vi "Tester.vi"() -> ()   [LabVIEW 2015]
uses:
  <resource>/Framework/Providers/lveio/public/EIOExtName.ctl
  <resource>/Framework/Providers/lveio/private/EIOResName.ctl
  <resource>/Framework/Providers/lveio/public/EIOResourceTree_TargetItem_GetProperty.vi
  <resource>/Framework/Providers/lveio/private/EIOResourceTree_TargetItem_GetResources.vi
  <resource>/Framework/Providers/lveio/public/EIOResourceTree_ProjectItem_GetDescendantNames.vi
panel:
  out "resources":T1[](array[typedef])
  out "value 2":string
  out "Array 3":string[](array[string])
  out "names":T2[](array[typedef])
  out "Tag:Get Names":string[](array[string])
  out "Array 2":string[](array[string])
  out "Array":string[](array[string])
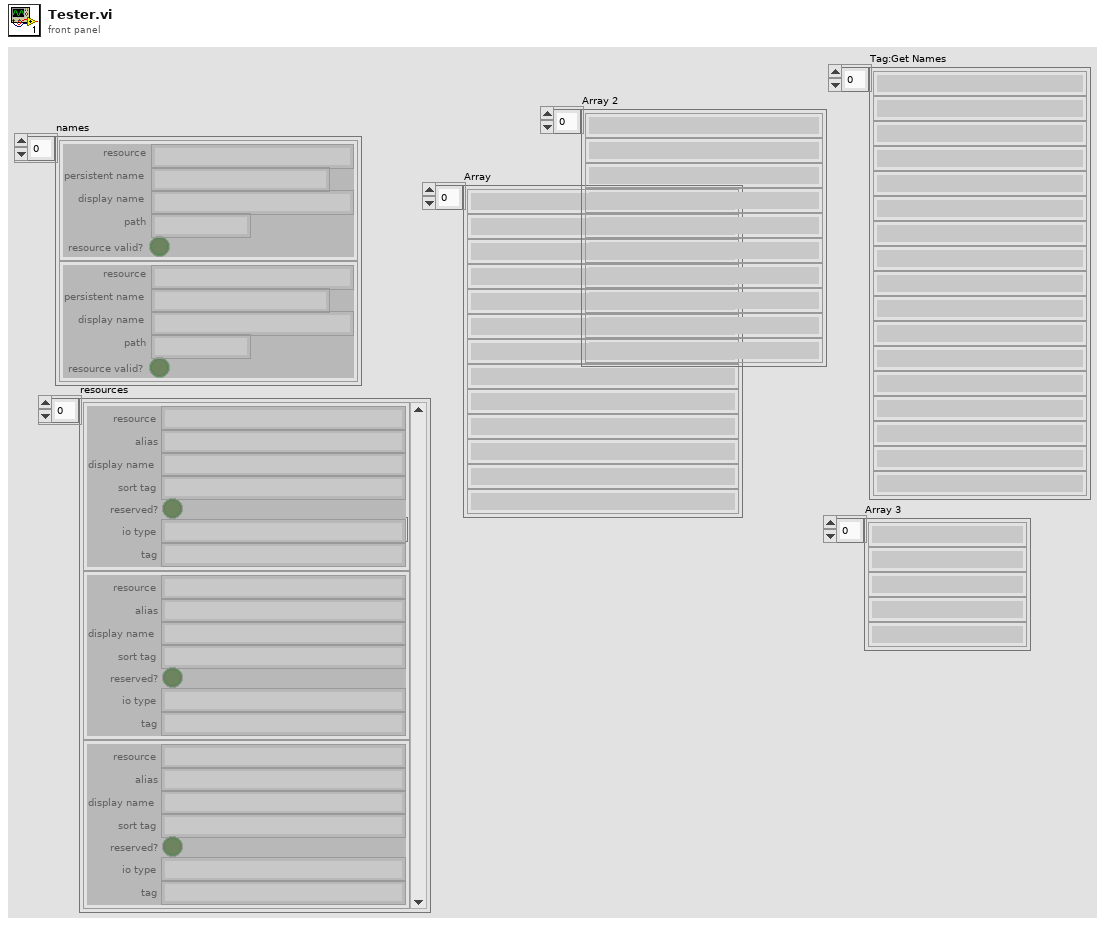
[diagram p1: front panel]
types:
  T1 = typedef "EIOResName.ctl" = cluster{"resource":string, "alias":string, "display name":string, "sort tag":string, "reserved?":bool, "io type":string, "tag":string}
  T2 = typedef "EIOExtName.ctl" = cluster{"resource":string, "persistent name":string, "display name":string, "path":string, "resource valid?":bool}
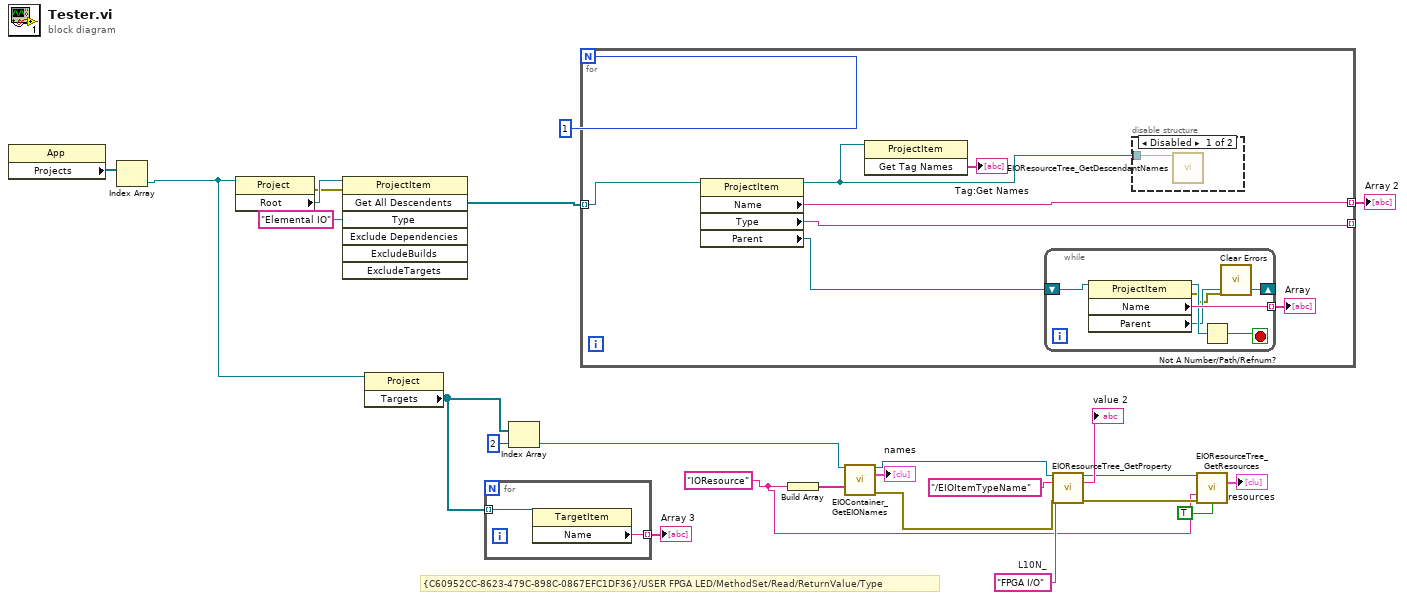
[diagram p0: block diagram]
diagram:
  w9 = "FPGA I/O"  # L10N_
  w3 = "IOResource" ("protocol")
  # "{C60952CC-8623-479C-898C-0867EFC1DF36}/USER FPGA LED/MethodSet/Read/ReturnValue/Type"
  n1 = property class="App"() -> ("Projects"=w24:refnum<vi>[])  [unwired: 2 in, 2 out]
  n2 = Index Array(array=w24) -> (element=w17:refnum<vi>)  [unwired: 1 in]
  n3 = property class="Project"(reference=w17) -> (error out=w22:errorcluster, "Root"=w23:refnum<vi>)  [unwired: 1 in, 1 out]
  n4 = invoke class="ProjectItem" method="Get All Descendents"(reference=w23, error in=w22, "Type"="Elemental IO") -> ("All Descendents"=w20:refnum<vi>[])  [unwired: 4 in, 6 out]
  n5 = property class="Project"(reference=w17) -> ("Targets"=w13:refnum<vi>[])  [unwired: 1 in, 2 out]
  n6 = for {
    tunnel: w13 -> [w26] mode=indexing
    tunnel: [w25] -> w11 mode=indexing
    n7 = property class="TargetItem"(reference=w26) -> ("Name"=w25:string)  [unwired: 1 in, 2 out]
  }
  "Array 3" <- w11
  n8 = Index Array(array=w13, index=2) -> (element=w12:refnum<vi>)
  n9 = for {
    N: 1 -> [_]
    tunnel: w20 -> [w33] mode=indexing
    tunnel: [w32] -> w18 mode=indexing
    tunnel: [w31] -> _ mode=indexing
    n10 = property class="ProjectItem"(reference=w33) -> (reference out=w28:refnum<vi>, "Name"=w32:string, "Type"=w31:string, "Parent"=w30:refnum<vi>)  [unwired: 1 in, 1 out]
    n11 = invoke class="ProjectItem" method="Get Tag Names"(reference=w28) -> ("Get Tag Names"=→"Tag:Get Names":string[])  [unwired: 2 in, 2 out]
    n12 = while {
      tunnel: [w39] -> w29 mode=indexing
      shift-right: [w36] -> _
      shift-left: w30 -> [w40]
      stop <- w37 stop-if-true
      n13 = property class="ProjectItem"(reference=w40) -> (reference out=w38:refnum<vi>, error out=w35:errorcluster, "Name"=w39:string, "Parent"=w36:refnum<vi>)  [unwired: 1 in]
      n14 = Not A Number/Path/Refnum?(number/path/refnum=w38) -> (NaN/Path/Refnum?=w37:bool)
      n15 = call <vilib>:"Clear Errors.vi"("error in (no error)"=w35) -> ()  [unwired: 5 in, 2 out]
    }
    "Array" <- w29
    n16 = disable-structure shown="Disabled" {
      disable-tunnel: w28 -> [w34 _]
      frame Disabled {
        n17 = call-poly <resource>:"EIOResourceTree_GetDescendantNames.vi"("Refnum In"=w34) -> ()  [unwired: 3 in, 12 out]
      }
      frame Enabled {
      }
    }
  }
  "Array 2" <- w18
  n18 = Build Array(w3) -> (w15:string[])
  n19 = call <resource>:"EIOContainer_GetEIONames.vi"("TargetItem Refnum In"=w12, "include protocols"=w15) -> ("TargetItem Refnum Out"=w8:refnum<vi>, "names"=→"names":T2[], "error out"=w7:errorcluster)  [unwired: 2 in, 9 out]
  n20 = call-poly <resource>:"EIOResourceTree_GetProperty.vi"("Refnum In"=w8, "property"="/EIOItemTypeName", "default value"=w9, "error in (no error)"=w7) -> ("Refnum Out"=w5:refnum<vi>, "value"=→"value 2":string, "error out"=w4:errorcluster)  [unwired: 9 out]
  n21 = call-poly <resource>:"EIOResourceTree_GetResources.vi"("Refnum In"=w5, "protocol"=w3, "error in (no error)"=w4, "Consider \"ExcludeFromUserSelections\" attribute (F)"=TRUE ("Consider \"ExcludeFromUserSelections\" attribute (F)")) -> ("resources"=→"resources":T1[])  [unwired: 1 in, 10 out]
